vi "Suite from Library.vi"(8 "error in (no error)":errorcluster, 10 "Library Path":path, 11 "LUnit Test Suite In":refnum<class "LUnit Test Suite.lvclass">) -> (0 "error out":errorcluster, 3 "LUnit Test Suite Out":refnum<class "LUnit Test Suite.lvclass">)   [LabVIEW 2020, in "Test Finder.lvclass"]
doc: "Produces a test suite from a .lvlib file."
uses:
  Test Finder.lvclass
  LUnit Test Suite.lvclass
  C:/git/astemes-lunit/source/Runnable.lvclass
  Private/Filter Test Cases.vi
  Private/Find all Classes in LV XML.vi
  <vilib>/Utility/LVClass/Get LV Class Default Value.vi
  LUnit Test Case.lvclass
  Test Finder.lvclass/Test Finder.ctl
  C:/git/astemes-lunit/source/LUnit Test Suite.lvclass
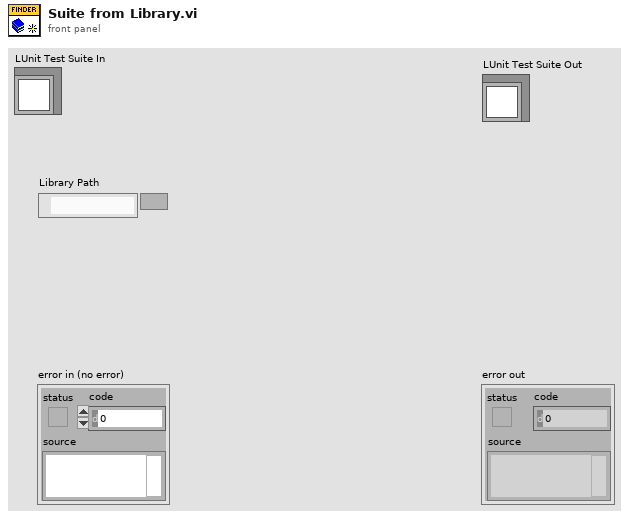
[diagram p1: front panel]
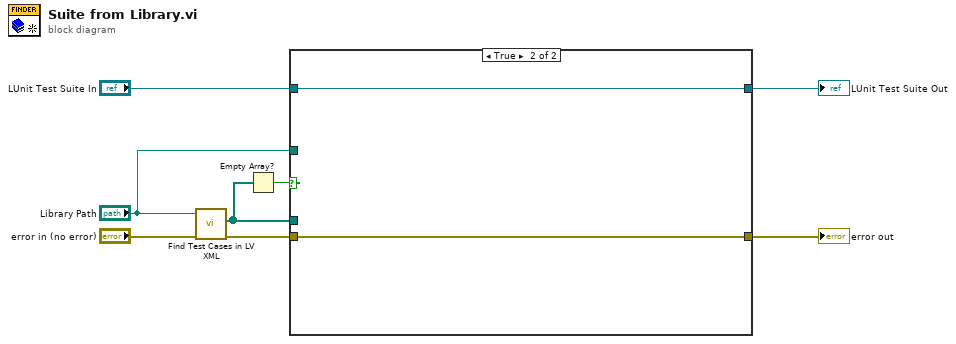
[diagram p0: block diagram]
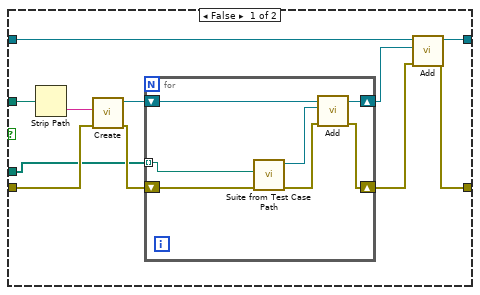
[diagram p2: hidden frame]
diagram:
  n1 = call "Find Test Cases in LV XML.vi"("error in (no error)"="error in (no error)", "Path"="Library Path") -> ("error out"=w4:errorcluster, "Test Class paths"=w3:path[])  [unwired: 8 in]
  n2 = Empty Array?(array=w3) -> (empty?=w2:bool)
  n3 = case shown="True" w2 {
    tunnel: [w19 w28] -> w7
    tunnel: "LUnit Test Suite In" -> [w18 w28]
    tunnel: [w16 w27] -> w5
    tunnel: w4 -> [w15 w27]
    tunnel: w3 -> [w11 _]
    tunnel: "Library Path" -> [w10 _]
    frame False {
      n4 = Strip Path(path=w10) -> (name=w9:string)  [unwired: 1 out]
      n5 = call "Create.vi"("error in (no error)"=w15, "Suite Name"=w9) -> ("error out"=w14:errorcluster, "LUnit Test Suite Out"=w13:refnum<class "LUnit Test Suite.lvclass">)  [unwired: 8 in]
      n6 = for {
        tunnel: w11 -> [w23] mode=indexing
        shift-right: [w26] -> w17
        shift-left: w14 -> [w22]
        shift-right: [w24] -> w12
        shift-left: w13 -> [w25]
        n7 = call "Suite from Test Case Path.vi"("error in (no error)"=w22, "Test Case"=w23) -> ("error out"=w21:errorcluster, "LUnit Test Suite Out"=w20:refnum<class "LUnit Test Suite.lvclass">)  [unwired: 8 in]
        n8 = call "Add.vi"("error in (no error)"=w21, "Runnable"=w20, "LUnit Test Suite In"=w25) -> ("error out"=w26:errorcluster, "LUnit Test Suite Out"=w24:refnum<class "LUnit Test Suite.lvclass">)  [unwired: 7 in]
      }
      n9 = call "Add.vi"("error in (no error)"=w17, "Runnable"=w12, "LUnit Test Suite In"=w18) -> ("error out"=w16:errorcluster, "LUnit Test Suite Out"=w19:refnum<class "LUnit Test Suite.lvclass">)  [unwired: 7 in]
    }
    frame True {
    }
  }
  "error out" <- w5
  "LUnit Test Suite Out" <- w7
